vi "GetPin.vi"(8 "error in (no error)":errorcluster, 9 "Pin":u8, 10 "Port":u8, 11 "Cypress CY8CKIT-059 in":refnum<class "Cypress CY8CKIT-059.lvclass">) -> (0 "error out":errorcluster, 1 "Response":string, 2 "Value":bool, 3 "Cypress CY8CKIT-059 out":refnum<class "Cypress CY8CKIT-059.lvclass">)   [LabVIEW 2020, in "Cypress CY8CKIT-059.lvclass"]
doc: "Sends a command to read the pin status from the target device."
uses:
  Cypress CY8CKIT-059.lvclass
  Controls/Device Code.ctl
  Controls/Device Command Code.ctl
  Cypress CY8CKIT-059.lvclass/Cypress CY8CKIT-059.ctl
  3342a513-f70f-4605-b988-32c53bdac969.vi
  Read Serial Port.vi
  Write Serial Port.vi
  <vilib>/Utility/error.llb/Error Cluster From Error Code.vi
  <vilib>/ErrorRing/Error Ring.xnode
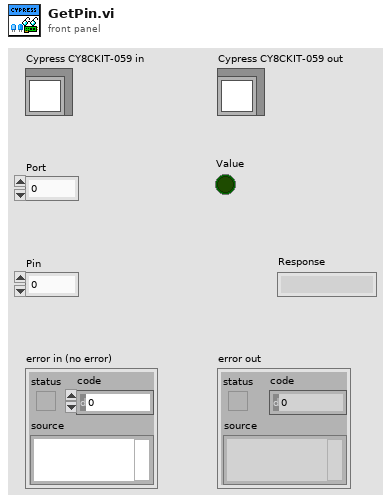
[diagram p1: front panel]
types:
  T1 = typedef "Device Command Code.ctl" = string
  T2 = typedef "Device Code.ctl" = string
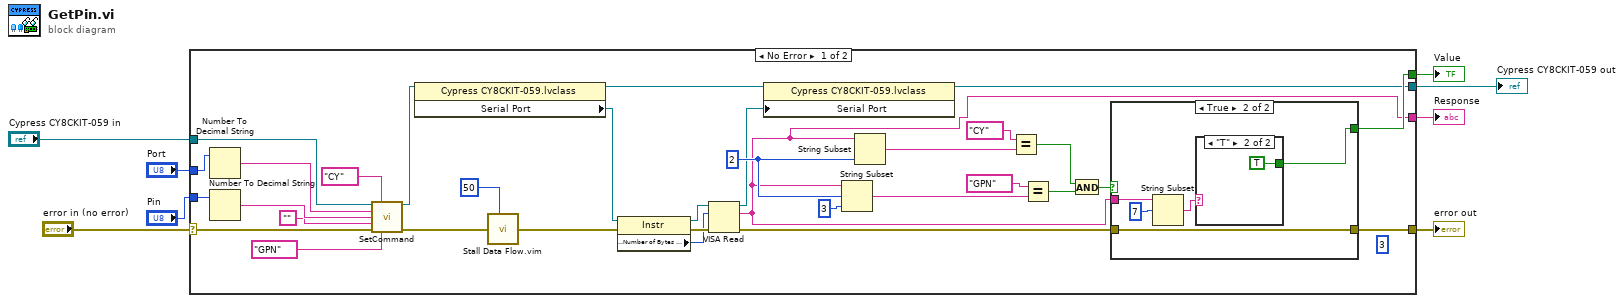
[diagram p0: block diagram]
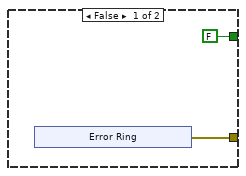
[diagram p2: hidden frame]
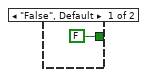
[diagram p3: hidden frame]
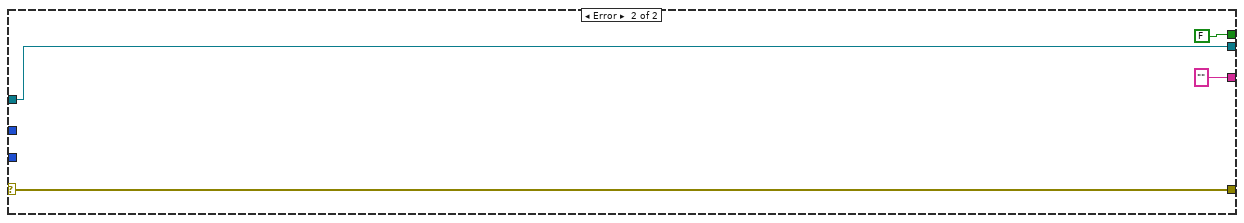
[diagram p4: hidden frame]
diagram:
  n1 = case shown="No Error" "error in (no error)" {
    selector: "error in (no error)" -> [w41 w58]
    tunnel: [w20 w58] -> w7
    tunnel: "Cypress CY8CKIT-059 in" -> [w39 w59]
    tunnel: [w15 w59] -> w5
    tunnel: "Port" -> [w37 _]
    tunnel: "Pin" -> [w35 _]
    tunnel: [w18 FALSE] -> w1
    tunnel: [w9 "" ("read buffer")] -> w2
    frame No Error {
      (unwired) 3 ("length (rest)")
      w26 = 2 ("length (rest)")
      n2 = Number To Decimal String(number=w37) -> (decimal integer string=w36:string)  [unwired: 1 in]
      n3 = Number To Decimal String(number=w35) -> (decimal integer string=w34:string)  [unwired: 1 in]
      n4 = call-dynamic "SetCommand.vi"("Cypress CY8CKIT-059 in"=w39, "Device Code"=T2 "CY", "Parameter 1"=w36, "Parameter 2"=w34, "Parameter 3"="", "error in (no error)"=w41, "Command Code"=T1 "GPN") -> ("Cypress CY8CKIT-059 out"=w32:refnum<class "Cypress CY8CKIT-059.lvclass">, "error out"=w12:errorcluster)  [unwired: 6 in, 1 out]
      n5 = property class="Cypress CY8CKIT-059.lvclass"(reference=w32) -> (reference out=w16:refnum<class "Cypress CY8CKIT-059.lvclass">, "Serial Port"=w31:refnum<visa-resource-name>)  [unwired: 1 in, 1 out]
      n6 = call "Stall Data Flow.vim"("value in"=w12, "milliseconds to wait"=u32 50) -> ("value out"=w11:errorcluster)  [unwired: 1 out]
      n7 = property class="Instr"(reference=w31, error in=w11) -> (reference out=w29:refnum<visa-resource-name>, error out=w30:errorcluster, "Serial Settings:Number of Bytes at Serial Port"=w28:u32)
      n8 = VISA Read(VISA resource name=w29, byte count=w28, error in (no error)=w30) -> (VISA resource name out=w14:refnum<visa-resource-name>, read buffer=w9:string, error out=w21:errorcluster)  [unwired: 1 out]
      n9 = property class="Cypress CY8CKIT-059.lvclass"(reference=w16, "Serial Port"=w14) -> (reference out=w15:refnum<class "Cypress CY8CKIT-059.lvclass">)  [unwired: 1 in, 1 out]
      n10 = String Subset(string=w9, offset (0)=w26, length (rest)=3 ("length (rest)")) -> (substring=w27:string)
      n11 = String Subset(string=w9, length (rest)=w26) -> (substring=w17:string)  [unwired: 1 in]
      n12 = Equal?(x=T2 "CY" ("Device Code"), y=w17) -> (x = y?=w19:bool)
      n13 = Equal?(x=T1 "GPN" ("Command Code"), y=w27) -> (x = y?=w23:bool)
      n14 = And(x=w19, y=w23) -> (x .and. y?=w22:bool)
      n15 = case shown="True" w22 {
        tunnel: w21 -> [_ w53]
        tunnel: [w43 w53] -> w20
        tunnel: w9 -> [_ w52]
        tunnel: [FALSE w49] -> w18
        frame False {
          n16 = xnode "Error Ring"() -> ("error out"=w43:errorcluster)
        }
        frame True {
          n17 = String Subset(string=w52, offset (0)=7) -> (substring=w50:string)  [unwired: 1 in]
          n18 = case shown="\"T\"" w50 {
            tunnel: [FALSE TRUE] -> w49
            frame "False", Default {
            }
            frame "T" {
            }
          }
        }
      }
    }
    frame Error {
    }
  }
  "error out" <- w7
  "Cypress CY8CKIT-059 out" <- w5
  "Response" <- w2
  "Value" <- w1
